vi "OEE_SCREEN_1_recolor.vi"(7 "SCREEN_1_recolor_references":T2, 8 "error_in":errorcluster, 11 "SCREEN_1":T1={"header_date"="-", "header_time"="-", "header_takt"="-", "header_shift"="-", "OP10_actual"="-", "OP10_rejects"="-", "OP10_quality_yeild"="-", "OP10_pace"="-", "OP20_actual"="-", "OP20_rejects"="-", "OP20_quality_yeild"="-", "OP20_pace"="-", "OP30_actual"="-", "OP30_rejects"="-", "OP30_quality_yeild"="-", "OP30_pace"="-", "OP40_actual"="-", "OP40_rejects"="-", "OP40_quality_yeild"="-", "OP40_pace"="-", "OP50_actual"="-", "OP50_rejects"="-", "OP50_quality_yeild"="-", "OP50_pace"="-", "OP60_actual"="-", "OP60_rejects"="-", "OP60_quality_yeild"="-", "OP60_pace"="-", "OP70_actual"="-", "OP70_rejects"="-", "OP70_quality_yeild"="-", "OP70_pace"="-", "OP80_actual"="-", "OP80_rejects"="-", "OP80_quality_yeild"="-", "OP80_pace"="-", "OP90_actual"="-", "OP90_rejects"="-", "OP90_quality_yeild"="-", "OP90_pace"="-", "OP100_actual"="-", "OP100_rejects"="-", "OP100_quality_yeild"="-", "OP100_pace"="-", "OP110_actual"="-", "OP110_rejects"="-", "OP110_quality_yeild"="-", "OP110_pace"="-", "OP120_actual"="-", "OP120_rejects"="-", "OP120_quality_yeild"="-", "OP120_pace"="-", "OP130_actual"="-", "OP130_rejects"="-", "OP130_quality_yeild"="-", "OP130_pace"="-", "OP10_header"="OP10", "OP20_header"="OP20", "OP30_header"="OP30", "OP40_header"="OP40", "OP50_header"="OP50", "OP60_header"="OP60", "OP70_header"="OP70", "OP80_header"="OP80", "OP90_header"="OP90", "OP100_header"="OP100", "OP110_header"="OP110", "OP120_header"="OP120", "OP130_header"="OP130", "additional_info"="", "bottleneck_OP"="-", "bottleneck_header"="LINE BOTTLENECK", "screen_1_header"="", "actual_header"="", "rejects_header"="", "FTTH_header"="", "pace_header"="", "actual_header"="", "rejects_header"="", "FTTH_header"="", "pace_header"=""}) -> (0 "error_out":errorcluster)   [LabVIEW 2019]
uses:
  typedef/SCREEN_1_recolor_references.ctl
  typedef/SCREEN_1.ctl
panel:
  # "OP"
  # "OP"
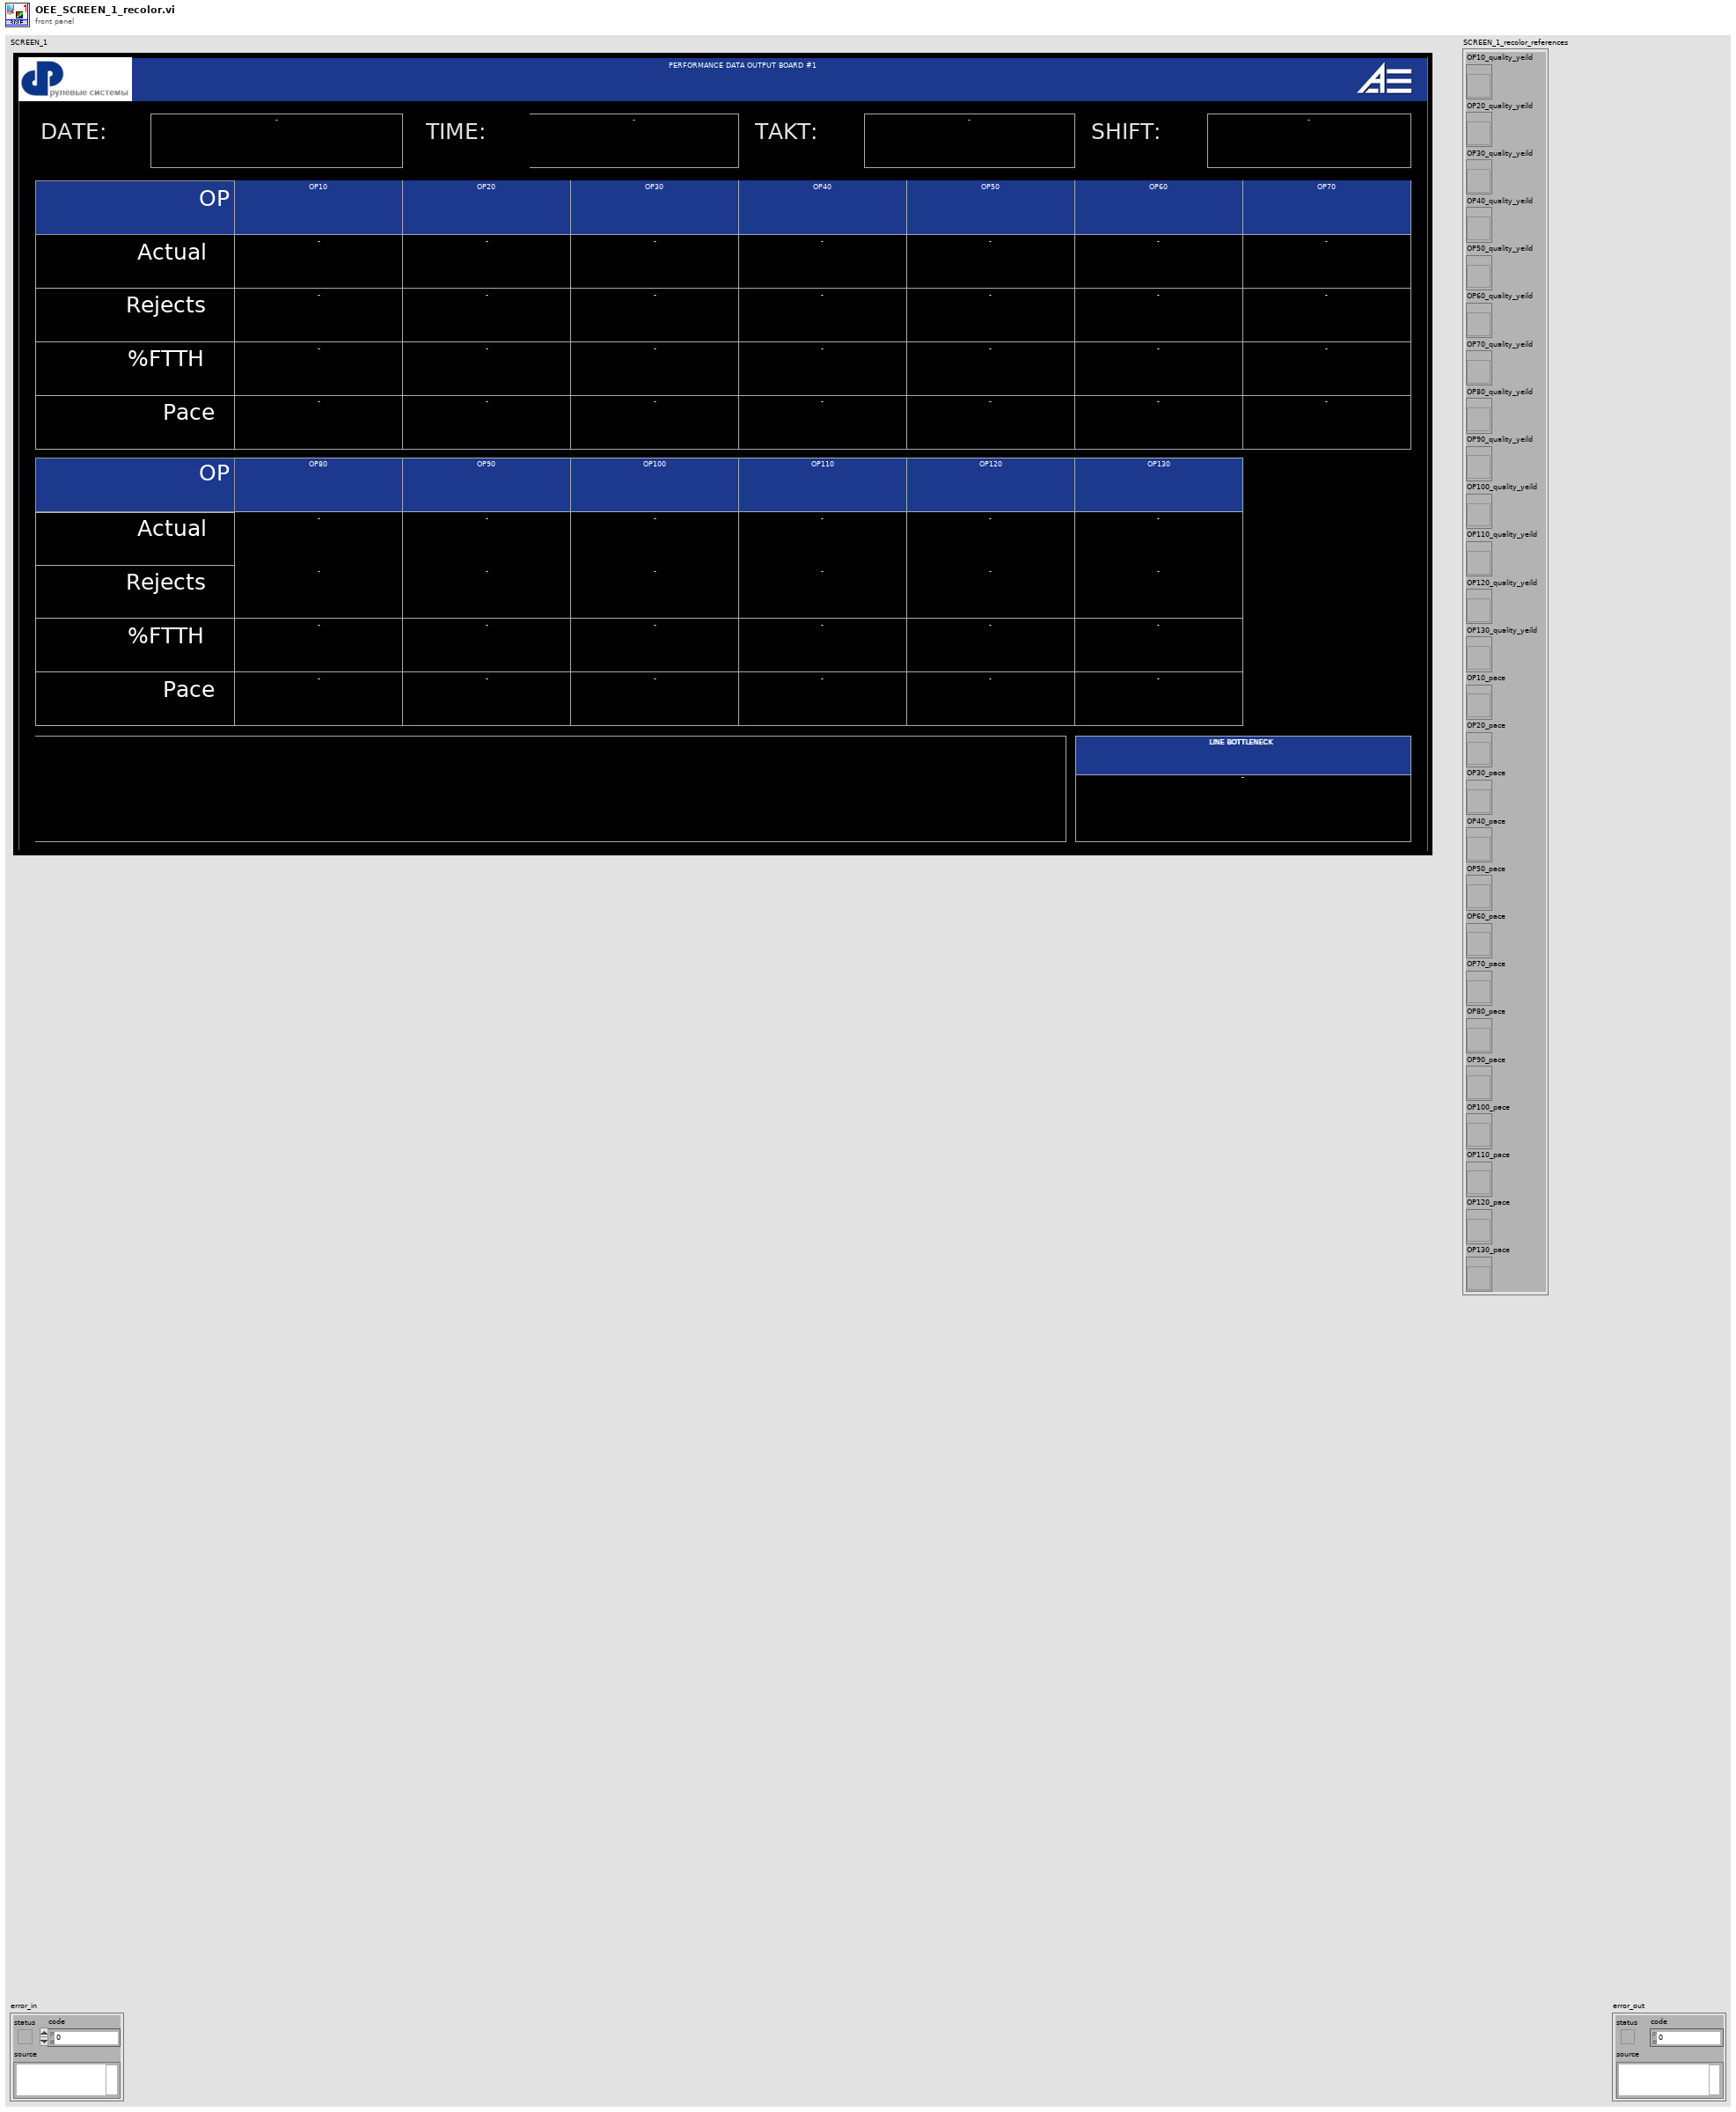
[diagram p1: front panel]
types:
  T1 = typedef "SCREEN_1.ctl" = cluster{"header_date":string, "header_time":string, "header_takt":string, "header_shift":string, "OP10_actual":string, "OP10_rejects":string, "OP10_quality_yeild":string, "OP10_pace":string, "OP20_actual":string, "OP20_rejects":string, "OP20_quality_yeild":string, "OP20_pace":string, "OP30_actual":string, "OP30_rejects":string, "OP30_quality_yeild":string, "OP30_pace":string, "OP40_actual":string, "OP40_rejects":string, "OP40_quality_yeild":string, "OP40_pace":string, "OP50_actual":string, "OP50_rejects":string, "OP50_quality_yeild":string, "OP50_pace":string, "OP60_actual":string, "OP60_rejects":string, "OP60_quality_yeild":string, "OP60_pace":string, "OP70_actual":string, "OP70_rejects":string, "OP70_quality_yeild":string, "OP70_pace":string, "OP80_actual":string, "OP80_rejects":string, "OP80_quality_yeild":string, "OP80_pace":string, "OP90_actual":string, "OP90_rejects":string, "OP90_quality_yeild":string, "OP90_pace":string, "OP100_actual":string, "OP100_rejects":string, "OP100_quality_yeild":string, "OP100_pace":string, "OP110_actual":string, "OP110_rejects":string, "OP110_quality_yeild":string, "OP110_pace":string, "OP120_actual":string, "OP120_rejects":string, "OP120_quality_yeild":string, "OP120_pace":string, "OP130_actual":string, "OP130_rejects":string, "OP130_quality_yeild":string, "OP130_pace":string, "OP10_header":string, "OP20_header":string, "OP30_header":string, "OP40_header":string, "OP50_header":string, "OP60_header":string, "OP70_header":string, "OP80_header":string, "OP90_header":string, "OP100_header":string, "OP110_header":string, "OP120_header":string, "OP130_header":string, "additional_info":string, "bottleneck_OP":string, "bottleneck_header":string, "screen_1_header":string, "actual_header":string, "rejects_header":string, "FTTH_header":string, "pace_header":string, "actual_header":string, "rejects_header":string, "FTTH_header":string, "pace_header":string}
  T2 = typedef "SCREEN_1_recolor_references.ctl" = cluster{"OP10_quality_yeild":refnum<vi>, "OP20_quality_yeild":refnum<vi>, "OP30_quality_yeild":refnum<vi>, "OP40_quality_yeild":refnum<vi>, "OP50_quality_yeild":refnum<vi>, "OP60_quality_yeild":refnum<vi>, "OP70_quality_yeild":refnum<vi>, "OP80_quality_yeild":refnum<vi>, "OP90_quality_yeild":refnum<vi>, "OP100_quality_yeild":refnum<vi>, "OP110_quality_yeild":refnum<vi>, "OP120_quality_yeild":refnum<vi>, "OP130_quality_yeild":refnum<vi>, "OP10_pace":refnum<vi>, "OP20_pace":refnum<vi>, "OP30_pace":refnum<vi>, "OP40_pace":refnum<vi>, "OP50_pace":refnum<vi>, "OP60_pace":refnum<vi>, "OP70_pace":refnum<vi>, "OP80_pace":refnum<vi>, "OP90_pace":refnum<vi>, "OP100_pace":refnum<vi>, "OP110_pace":refnum<vi>, "OP120_pace":refnum<vi>, "OP130_pace":refnum<vi>}
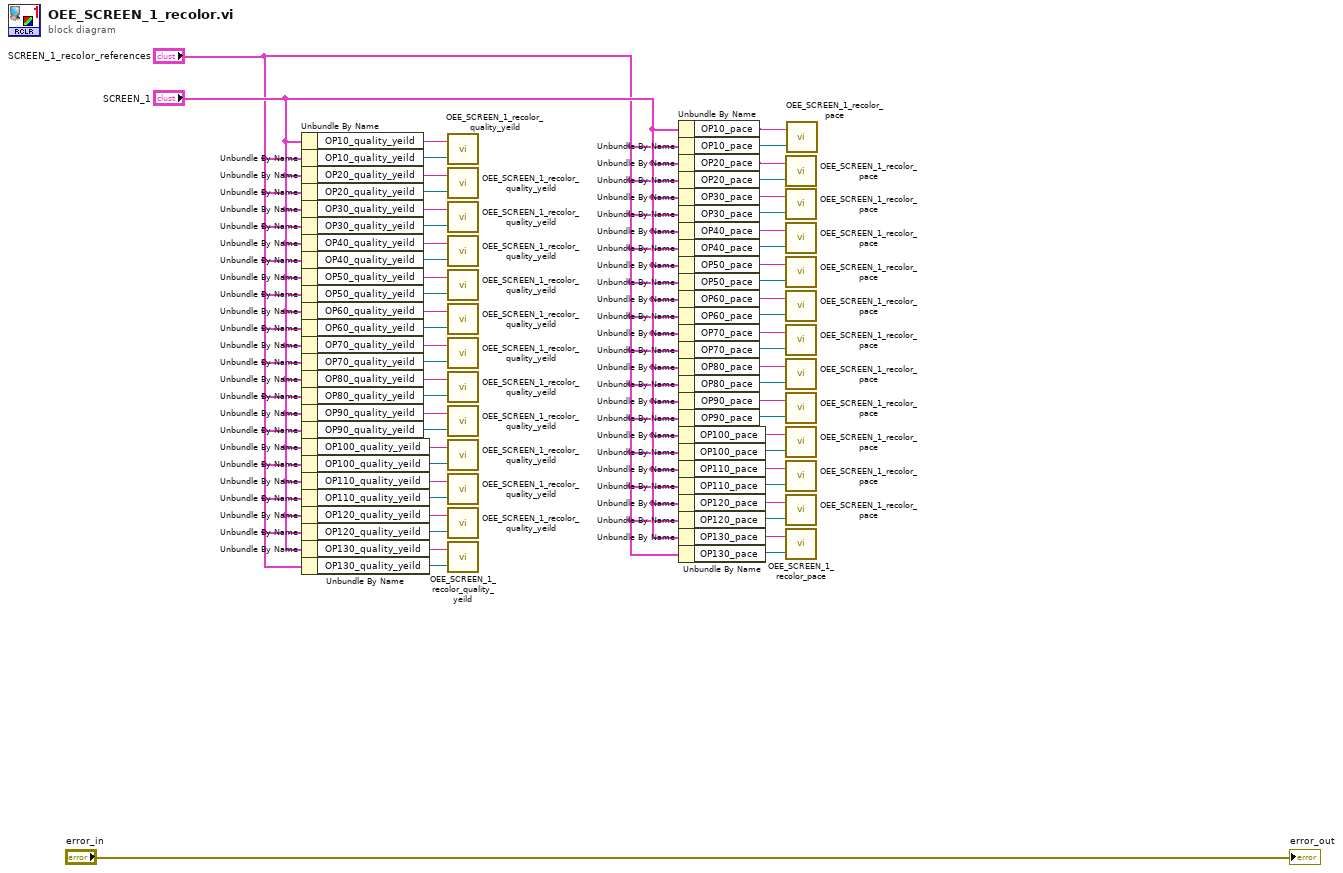
[diagram p0: block diagram]
diagram:
  n1 = Unbundle By Name("SCREEN_1") -> ("OP10_quality_yeild"=w55:string)
  n2 = Unbundle By Name("SCREEN_1_recolor_references") -> ("OP10_quality_yeild"=w54:refnum<vi>)
  n3 = Unbundle By Name("SCREEN_1") -> ("OP20_quality_yeild"=w53:string)
  n4 = Unbundle By Name("SCREEN_1_recolor_references") -> ("OP20_quality_yeild"=w52:refnum<vi>)
  n5 = Unbundle By Name("SCREEN_1") -> ("OP30_quality_yeild"=w51:string)
  n6 = Unbundle By Name("SCREEN_1_recolor_references") -> ("OP30_quality_yeild"=w50:refnum<vi>)
  n7 = Unbundle By Name("SCREEN_1") -> ("OP40_quality_yeild"=w47:string)
  n8 = Unbundle By Name("SCREEN_1_recolor_references") -> ("OP40_quality_yeild"=w46:refnum<vi>)
  n9 = Unbundle By Name("SCREEN_1") -> ("OP50_quality_yeild"=w45:string)
  n10 = Unbundle By Name("SCREEN_1_recolor_references") -> ("OP50_quality_yeild"=w44:refnum<vi>)
  n11 = Unbundle By Name("SCREEN_1") -> ("OP60_quality_yeild"=w43:string)
  n12 = Unbundle By Name("SCREEN_1_recolor_references") -> ("OP60_quality_yeild"=w42:refnum<vi>)
  n13 = Unbundle By Name("SCREEN_1") -> ("OP70_quality_yeild"=w41:string)
  n14 = Unbundle By Name("SCREEN_1_recolor_references") -> ("OP70_quality_yeild"=w40:refnum<vi>)
  n15 = Unbundle By Name("SCREEN_1") -> ("OP80_quality_yeild"=w39:string)
  n16 = Unbundle By Name("SCREEN_1_recolor_references") -> ("OP80_quality_yeild"=w38:refnum<vi>)
  n17 = Unbundle By Name("SCREEN_1") -> ("OP90_quality_yeild"=w37:string)
  n18 = Unbundle By Name("SCREEN_1_recolor_references") -> ("OP90_quality_yeild"=w36:refnum<vi>)
  n19 = Unbundle By Name("SCREEN_1") -> ("OP100_quality_yeild"=w35:string)
  n20 = Unbundle By Name("SCREEN_1_recolor_references") -> ("OP100_quality_yeild"=w34:refnum<vi>)
  n21 = Unbundle By Name("SCREEN_1") -> ("OP110_quality_yeild"=w33:string)
  n22 = Unbundle By Name("SCREEN_1_recolor_references") -> ("OP110_quality_yeild"=w32:refnum<vi>)
  n23 = Unbundle By Name("SCREEN_1") -> ("OP120_quality_yeild"=w31:string)
  n24 = Unbundle By Name("SCREEN_1_recolor_references") -> ("OP120_quality_yeild"=w30:refnum<vi>)
  n25 = Unbundle By Name("SCREEN_1") -> ("OP130_quality_yeild"=w49:string)
  n26 = Unbundle By Name("SCREEN_1_recolor_references") -> ("OP130_quality_yeild"=w48:refnum<vi>)
  n27 = call "OEE_SCREEN_1_recolor_quality_yeild.vi"("quality_yeild_field_reference"=w54, "quality_yeild_value"=w55) -> ()  [unwired: 1 in]
  n28 = call "OEE_SCREEN_1_recolor_quality_yeild.vi"("quality_yeild_field_reference"=w52, "quality_yeild_value"=w53) -> ()  [unwired: 1 in]
  n29 = call "OEE_SCREEN_1_recolor_quality_yeild.vi"("quality_yeild_field_reference"=w50, "quality_yeild_value"=w51) -> ()  [unwired: 1 in]
  n30 = call "OEE_SCREEN_1_recolor_quality_yeild.vi"("quality_yeild_field_reference"=w46, "quality_yeild_value"=w47) -> ()  [unwired: 1 in]
  n31 = call "OEE_SCREEN_1_recolor_quality_yeild.vi"("quality_yeild_field_reference"=w44, "quality_yeild_value"=w45) -> ()  [unwired: 1 in]
  n32 = call "OEE_SCREEN_1_recolor_quality_yeild.vi"("quality_yeild_field_reference"=w42, "quality_yeild_value"=w43) -> ()  [unwired: 1 in]
  n33 = call "OEE_SCREEN_1_recolor_quality_yeild.vi"("quality_yeild_field_reference"=w40, "quality_yeild_value"=w41) -> ()  [unwired: 1 in]
  n34 = call "OEE_SCREEN_1_recolor_quality_yeild.vi"("quality_yeild_field_reference"=w38, "quality_yeild_value"=w39) -> ()  [unwired: 1 in]
  n35 = call "OEE_SCREEN_1_recolor_quality_yeild.vi"("quality_yeild_field_reference"=w36, "quality_yeild_value"=w37) -> ()  [unwired: 1 in]
  n36 = call "OEE_SCREEN_1_recolor_quality_yeild.vi"("quality_yeild_field_reference"=w34, "quality_yeild_value"=w35) -> ()  [unwired: 1 in]
  n37 = call "OEE_SCREEN_1_recolor_quality_yeild.vi"("quality_yeild_field_reference"=w32, "quality_yeild_value"=w33) -> ()  [unwired: 1 in]
  n38 = call "OEE_SCREEN_1_recolor_quality_yeild.vi"("quality_yeild_field_reference"=w30, "quality_yeild_value"=w31) -> ()  [unwired: 1 in]
  n39 = call "OEE_SCREEN_1_recolor_quality_yeild.vi"("quality_yeild_field_reference"=w48, "quality_yeild_value"=w49) -> ()  [unwired: 1 in]
  n40 = Unbundle By Name("SCREEN_1") -> ("OP10_pace"=w28:string)
  n41 = Unbundle By Name("SCREEN_1_recolor_references") -> ("OP10_pace"=w27:refnum<vi>)
  n42 = Unbundle By Name("SCREEN_1") -> ("OP20_pace"=w21:string)
  n43 = Unbundle By Name("SCREEN_1_recolor_references") -> ("OP20_pace"=w24:refnum<vi>)
  n44 = Unbundle By Name("SCREEN_1") -> ("OP30_pace"=w20:string)
  n45 = Unbundle By Name("SCREEN_1_recolor_references") -> ("OP30_pace"=w19:refnum<vi>)
  n46 = Unbundle By Name("SCREEN_1") -> ("OP40_pace"=w18:string)
  n47 = Unbundle By Name("SCREEN_1_recolor_references") -> ("OP40_pace"=w17:refnum<vi>)
  n48 = Unbundle By Name("SCREEN_1") -> ("OP50_pace"=w16:string)
  n49 = Unbundle By Name("SCREEN_1_recolor_references") -> ("OP50_pace"=w15:refnum<vi>)
  n50 = Unbundle By Name("SCREEN_1") -> ("OP60_pace"=w14:string)
  n51 = Unbundle By Name("SCREEN_1_recolor_references") -> ("OP60_pace"=w13:refnum<vi>)
  n52 = Unbundle By Name("SCREEN_1") -> ("OP70_pace"=w12:string)
  n53 = Unbundle By Name("SCREEN_1_recolor_references") -> ("OP70_pace"=w11:refnum<vi>)
  n54 = Unbundle By Name("SCREEN_1") -> ("OP80_pace"=w10:string)
  n55 = Unbundle By Name("SCREEN_1_recolor_references") -> ("OP80_pace"=w9:refnum<vi>)
  n56 = Unbundle By Name("SCREEN_1") -> ("OP90_pace"=w8:string)
  n57 = Unbundle By Name("SCREEN_1_recolor_references") -> ("OP90_pace"=w7:refnum<vi>)
  n58 = Unbundle By Name("SCREEN_1") -> ("OP100_pace"=w6:string)
  n59 = Unbundle By Name("SCREEN_1_recolor_references") -> ("OP100_pace"=w5:refnum<vi>)
  n60 = Unbundle By Name("SCREEN_1") -> ("OP110_pace"=w4:string)
  n61 = Unbundle By Name("SCREEN_1_recolor_references") -> ("OP110_pace"=w3:refnum<vi>)
  n62 = Unbundle By Name("SCREEN_1") -> ("OP120_pace"=w2:string)
  n63 = Unbundle By Name("SCREEN_1_recolor_references") -> ("OP120_pace"=w1:refnum<vi>)
  n64 = Unbundle By Name("SCREEN_1") -> ("OP130_pace"=w23:string)
  n65 = Unbundle By Name("SCREEN_1_recolor_references") -> ("OP130_pace"=w22:refnum<vi>)
  n66 = call "OEE_SCREEN_1_recolor_pace.vi"("pace_field_reference"=w24, "pace_value"=w21) -> ()  [unwired: 1 in]
  n67 = call "OEE_SCREEN_1_recolor_pace.vi"("pace_field_reference"=w19, "pace_value"=w20) -> ()  [unwired: 1 in]
  n68 = call "OEE_SCREEN_1_recolor_pace.vi"("pace_field_reference"=w17, "pace_value"=w18) -> ()  [unwired: 1 in]
  n69 = call "OEE_SCREEN_1_recolor_pace.vi"("pace_field_reference"=w15, "pace_value"=w16) -> ()  [unwired: 1 in]
  n70 = call "OEE_SCREEN_1_recolor_pace.vi"("pace_field_reference"=w13, "pace_value"=w14) -> ()  [unwired: 1 in]
  n71 = call "OEE_SCREEN_1_recolor_pace.vi"("pace_field_reference"=w11, "pace_value"=w12) -> ()  [unwired: 1 in]
  n72 = call "OEE_SCREEN_1_recolor_pace.vi"("pace_field_reference"=w9, "pace_value"=w10) -> ()  [unwired: 1 in]
  n73 = call "OEE_SCREEN_1_recolor_pace.vi"("pace_field_reference"=w7, "pace_value"=w8) -> ()  [unwired: 1 in]
  n74 = call "OEE_SCREEN_1_recolor_pace.vi"("pace_field_reference"=w5, "pace_value"=w6) -> ()  [unwired: 1 in]
  n75 = call "OEE_SCREEN_1_recolor_pace.vi"("pace_field_reference"=w3, "pace_value"=w4) -> ()  [unwired: 1 in]
  n76 = call "OEE_SCREEN_1_recolor_pace.vi"("pace_field_reference"=w1, "pace_value"=w2) -> ()  [unwired: 1 in]
  n77 = call "OEE_SCREEN_1_recolor_pace.vi"("pace_field_reference"=w22, "pace_value"=w23) -> ()  [unwired: 1 in]
  n78 = call "OEE_SCREEN_1_recolor_pace.vi"("pace_field_reference"=w27, "pace_value"=w28) -> ()  [unwired: 1 in]
  "error_out" <- "error_in"
